vi "test - Generate Assert VI Template Path - U16.vi"(8 "error in (no error)":errorcluster, 11 "TestCase in":refnum<class "Create New Assert Tester.lvclass">) -> (0 "error out":errorcluster, 3 "TestCase out":refnum<class "Create New Assert Tester.lvclass">)   [LabVIEW 2016, in "Create New Assert Tester.lvclass"]
uses:
  Create New Assert Tester.lvclass
  <vilib>/Utility/Data Type/Type Definitions/Data Type.ctl
  <vilib>/addons/_JKI Toolkits/VI Tester/TestCase.llb/TestCase.lvclass
  <vilib>/Utility/Data Type/NI_Data Type.lvlib
  C:/Program Files (x86)/National Instruments/LabVIEW 2016/vi.lib/addons/_JKI Toolkits/VI Tester/TestCase.llb/TestCase.lvclass
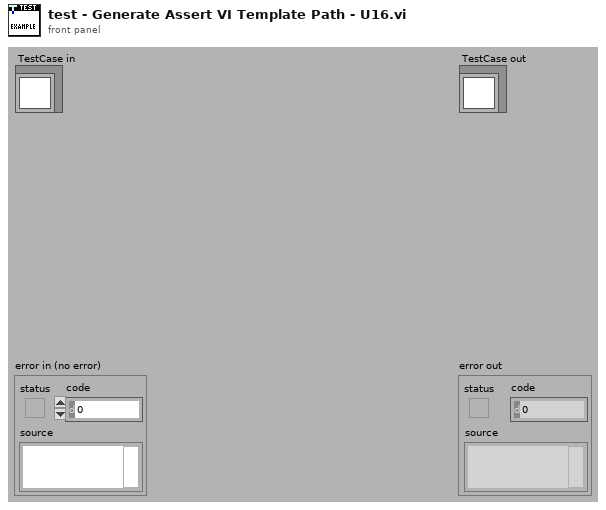
[diagram p1: front panel]
types:
  T1 = typedef "NI_Data Type.lvlib/Data Type.ctl" = enum8{"Invalid Type", "Void", "I8", "I16", "I32", "I64", "U8", "U16", "U32", "U64", "Single Float", "Double Float", "Extended Float", "Single Complex", "Double Complex", "Extended Complex", "Enum U8", "Enum U16", "Enum U32", "Enum U64", "Single Float With Unit", "Double Float With Unit", "Extended Float With Unit", "Single Complex with Unit", "Double Complex with Unit", "Extended Complex with Unit", "Boolean", "String", "Path", "Picture", "Tag", "Array", "Cluster", "Variant", "LV Variant", "Waveform", "Timestamp", "Digital Waveform", "Digital Data", "ExpressData", "Refnum", "External Data", "VI", "Poly VI", "LabVIEW Class Instance", "Fixed Point"}
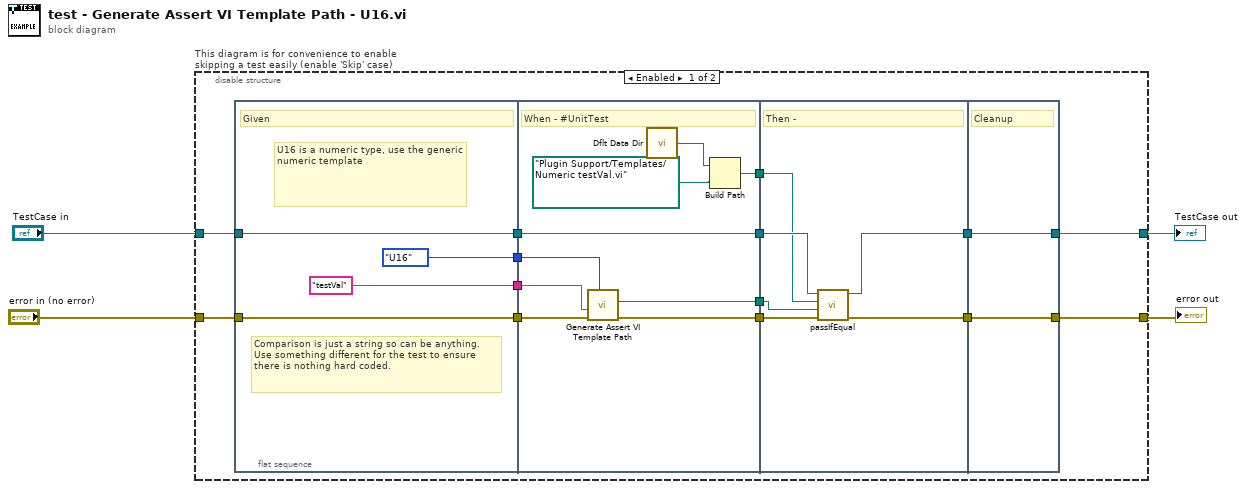
[diagram p0: block diagram]
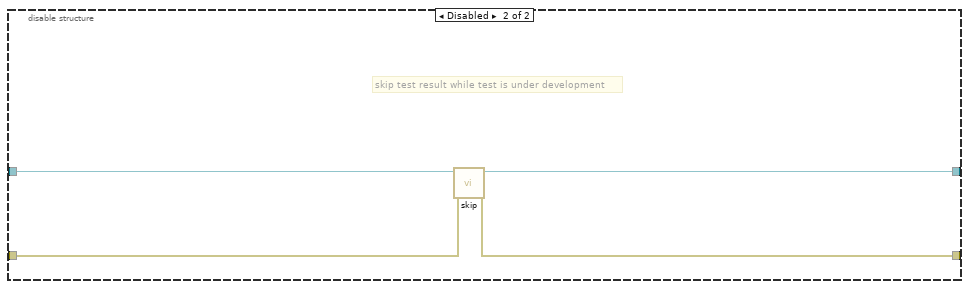
[diagram p2: hidden frame]
diagram:
  n1 = disable-structure "This diagram is for convenience to enable skipping a test easily (enable 'Skip' case)" shown="Enabled" {
    disable-tunnel: "TestCase in" -> [w12 w43]
    disable-tunnel: [w9 w41] -> w1
    disable-tunnel: [w10 w42] -> w3
    disable-tunnel: "error in (no error)" -> [w11 w40]
    frame Enabled {
      n2 = flat-sequence {
        tunnel: w11 -> [w21]
        tunnel: w12 -> [w22]
        tunnel: [w22] -> w18
        tunnel: [w21] -> w17
        tunnel: [Data_Type."U16" ("Data Type")] -> w8
        tunnel: ["testVal" ("Operation")] -> w7
        tunnel: [w31] -> w16
        tunnel: [w29] -> w15
        tunnel: w18 -> [w31]
        tunnel: w17 -> [w30]
        tunnel: w8 -> [w28]
        tunnel: w7 -> [w27]
        tunnel: [w26] -> w6
        tunnel: [w23] -> w5
        tunnel: [w34] -> w14
        tunnel: [w36] -> w13
        tunnel: w16 -> [w35]
        tunnel: w15 -> [w37]
        tunnel: w6 -> [w33]
        tunnel: w5 -> [w32]
        tunnel: [w38] -> w10
        tunnel: [w39] -> w9
        tunnel: w14 -> [w39]
        tunnel: w13 -> [w38]
        frame #0 {
          # "Comparison is just a string so can be anything. Use something different for the test to ensure there is nothing hard coded."
          # "U16 is a numeric type, use the generic numeric template"
          # "Given"
        }
        frame #1 {
          # "When - #UnitTest"
          n3 = call "Generate Assert VI Template Path.vi"("Data Type"=w28, "error in (no error)"=w30, "Operation"=w27) -> ("error out"=w29:errorcluster, "Template Path"=w26:path)  [unwired: 7 in]
          n4 = call <vilib>:"Dflt Data Dir.vi"() -> ("App:Default Data Directory"=w24:path)
          n5 = Build Path(base path=w24, name or relative path=path "Plugin Support/Templates/Numeric testVal.vi") -> (appended path=w23:path)
        }
        frame #2 {
          # "Then -"
          n6 = call-dynamic "passIfEqual.vi"("error in (no error)"=w37, "y"=w33, "x"=w32, "TestCase in"=w35) -> ("error out"=w36:errorcluster, "TestCase out"=w34:refnum<class "Create New Assert Tester.lvclass">)  [unwired: 6 in]
        }
        frame #3 {
          # "Cleanup"
        }
      }
    }
    frame Disabled {
      # "skip test result while test is under development"
      n7 = call <vilib>:"skip.vi"("error in (no error)"=w40, "TestCase in"=w43) -> ("error out"=w42:errorcluster, "TestCase out"=w41:refnum<class "Create New Assert Tester.lvclass">)  [unwired: 8 in]
    }
  }
  "error out" <- w3
  "TestCase out" <- w1
